vi "Check and update pretomo counters.vi"(8 "error in (no error)":errorcluster, 11 "Tomo in":refnum<class "Tomo.lvclass">) -> (0 "error out":errorcluster, 1 "continue stack?":bool, 2 "continue acquiring?":bool, 3 "Tomo out":refnum<class "Tomo.lvclass">)   [LabVIEW 2012, in "Tomo.lvclass"]
uses:
  Tomo.lvclass
  Tomo.lvclass/Tomo.ctl
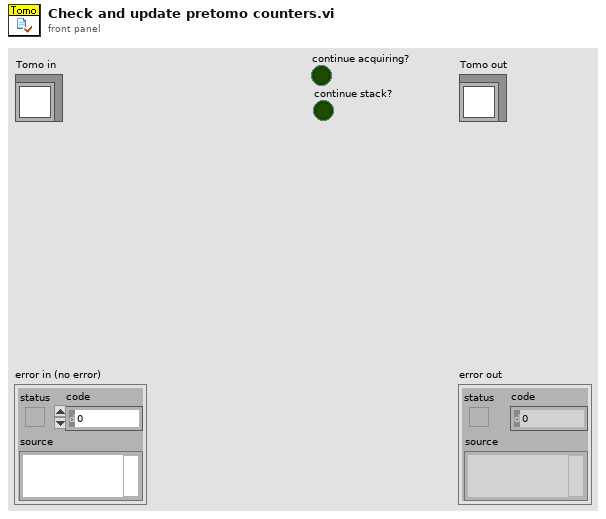
[diagram p1: front panel]
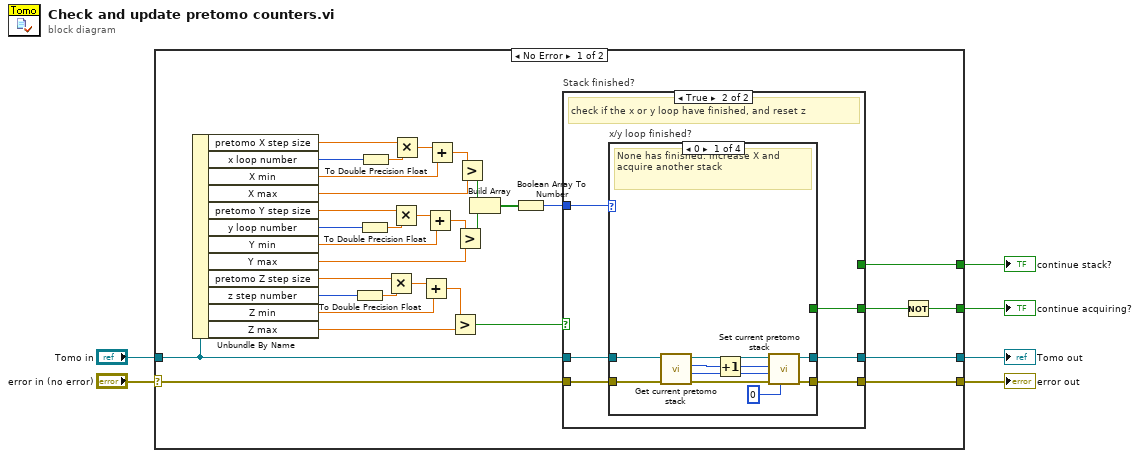
[diagram p0: block diagram]
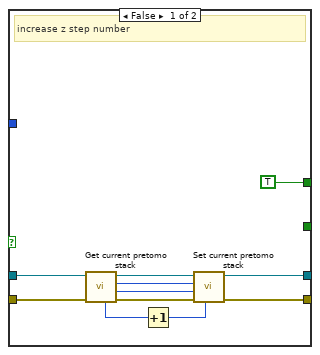
[diagram p2: hidden frame]
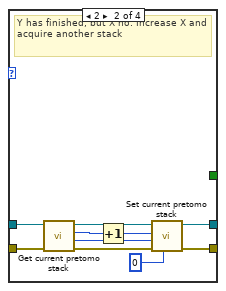
[diagram p3: hidden frame]
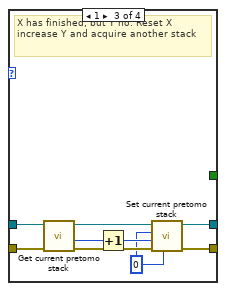
[diagram p4: hidden frame]
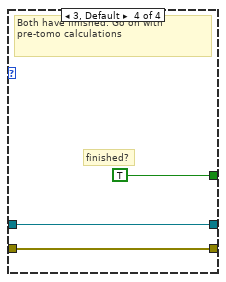
[diagram p5: hidden frame]
diagram:
  n1 = case shown="No Error" "error in (no error)" {
    selector: "error in (no error)" -> [w23 w90]
    tunnel: [w20 w90] -> w5
    tunnel: [w21 w89] -> w3
    tunnel: "Tomo in" -> [w22 w89]
    tunnel: [w18 _] -> w2
    tunnel: [w9 _] -> w1
    frame No Error {
      n2 = Unbundle By Name(w22) -> ("pretomo X step size"=w39:dbl[unit], "x loop number"=w8:i32, "X min"=w37:dbl[unit], "X max"=w35:dbl[unit], "pretomo Y step size"=w29:dbl[unit], "y loop number"=w7:i32, "Y min"=w30:dbl[unit], "Y max"=w28:dbl[unit], "pretomo Z step size"=w17:dbl[unit], "z step number"=w16:i32, "Z min"=w14:dbl[unit], "Z max"=w12:dbl[unit])
      n3 = To Double Precision Float(number=w16) -> (double precision float=w15:dbl)
      n4 = To Double Precision Float(number=w7) -> (double precision float=w33:dbl)
      n5 = To Double Precision Float(number=w8) -> (double precision float=w38:dbl)
      n6 = Multiply(x=w17, y=w15) -> (x*y=w13:dbl[unit])
      n7 = Multiply(x=w29, y=w33) -> (x*y=w32:dbl[unit])
      n8 = Multiply(x=w39, y=w38) -> (x*y=w36:dbl[unit])
      n9 = Add(x=w13, y=w14) -> (x+y=w11:dbl[unit])
      n10 = Add(x=w32, y=w30) -> (x+y=w31:dbl[unit])
      n11 = Add(x=w36, y=w37) -> (x+y=w34:dbl[unit])
      n12 = Greater?(x=w11, y=w12) -> (0:w10:bool)
      n13 = Greater?(x=w31, y=w28) -> (0:w26:bool)
      n14 = Greater?(x=w34, y=w35) -> (0:w27:bool)
      n15 = Build Array(w27, w26) -> (w25:bool[])
      n16 = Boolean Array To Number(Boolean array=w25) -> (number=w24:u32)
      n17 = case "Stack finished?" shown="True" w10 {
        tunnel: w24 -> [_ w56]
        tunnel: w23 -> [w47 w55]
        tunnel: w22 -> [w48 w54]
        tunnel: [w46 w53] -> w21
        tunnel: [w45 w52] -> w20
        tunnel: [_ w51] -> w19
        tunnel: [TRUE _] -> w9
        frame False {
          # "increase z step number"
          n18 = call-dynamic "Get current pretomo stack.vi"("error in (no error)"=w47, "Tomo in"=w48) -> ("error out"=w50:errorcluster, "y loop number"=w43:i32, "x loop number"=w44:i32, "Tomo out"=w49:refnum<class "Tomo.lvclass">, "z step number"=w42:i32)  [unwired: 5 in]
          n19 = Increment(x=w42) -> (x+1=w41:i32)
          n20 = call-dynamic "Set current pretomo stack.vi"("z step number"=w41, "error in (no error)"=w50, "current y stack"=w43, "current x stack"=w44, "Tomo in"=w49) -> ("error out"=w45:errorcluster, "Tomo out"=w46:refnum<class "Tomo.lvclass">)  [unwired: 5 in]
        }
        frame True {
          # "check if the x or y loop have finished, and reset z"
          n21 = case "x/y loop finished?" shown="0" w56 {
            tunnel: w55 -> [w66 w70 w82 w87]
            tunnel: w54 -> [w65 w71 w83 w88]
            tunnel: [w59 w69 w79 w88] -> w53
            tunnel: [w58 w68 w78 w87] -> w52
            tunnel: [_ _ _ TRUE] -> w51
            frame 0 {
              # "None has finished. Increase X and acquire another stack"
              n22 = call-dynamic "Get current pretomo stack.vi"("error in (no error)"=w66, "Tomo in"=w65) -> ("error out"=w63:errorcluster, "y loop number"=w60:i32, "x loop number"=w64:i32, "Tomo out"=w62:refnum<class "Tomo.lvclass">)  [unwired: 5 in, 1 out]
              n23 = Increment(x=w64) -> (x+1=w61:i32)
              n24 = call-dynamic "Set current pretomo stack.vi"("z step number"=0, "error in (no error)"=w63, "current y stack"=w60, "current x stack"=w61, "Tomo in"=w62) -> ("error out"=w58:errorcluster, "Tomo out"=w59:refnum<class "Tomo.lvclass">)  [unwired: 5 in]
            }
            frame 2 {
              # "Y has finished, but X no. Increase X and acquire another stack"
              n25 = call-dynamic "Get current pretomo stack.vi"("error in (no error)"=w70, "Tomo in"=w71) -> ("error out"=w73:errorcluster, "y loop number"=w76:i32, "x loop number"=w72:i32, "Tomo out"=w74:refnum<class "Tomo.lvclass">)  [unwired: 5 in, 1 out]
              n26 = Increment(x=w72) -> (x+1=w75:i32)
              n27 = call-dynamic "Set current pretomo stack.vi"("z step number"=0, "error in (no error)"=w73, "current y stack"=w76, "current x stack"=w75, "Tomo in"=w74) -> ("error out"=w68:errorcluster, "Tomo out"=w69:refnum<class "Tomo.lvclass">)  [unwired: 5 in]
            }
            frame 1 {
              w77 = 0 ("current x stack")
              # "X has finished, but Y no. Reset X  increase Y and acquire another stack"
              n28 = call-dynamic "Get current pretomo stack.vi"("error in (no error)"=w82, "Tomo in"=w83) -> ("error out"=w85:errorcluster, "y loop number"=w81:i32, "Tomo out"=w84:refnum<class "Tomo.lvclass">)  [unwired: 5 in, 2 out]
              n29 = Increment(x=w81) -> (x+1=w80:i32)
              n30 = call-dynamic "Set current pretomo stack.vi"("z step number"=w77, "error in (no error)"=w85, "current y stack"=w80, "current x stack"=w77, "Tomo in"=w84) -> ("error out"=w78:errorcluster, "Tomo out"=w79:refnum<class "Tomo.lvclass">)  [unwired: 5 in]
            }
            frame 3, Default {
              # "finished?"
              # "Both have finished. Go on with pre-tomo calculations"
            }
          }
        }
      }
      n31 = Not(x=w19) -> (.not. x?=w18:bool)
    }
    frame Error {
    }
  }
  "error out" <- w5
  "Tomo out" <- w3
  "continue acquiring?" <- w2
  "continue stack?" <- w1
